vi "stacked secuence.vi"() -> ()   [LabVIEW 2020]
panel:
  out "Boolean":bool
  in  "Button":bool
  out "Thermometer":u8(slide) scale=0.0..100.0
  in  "stop":bool
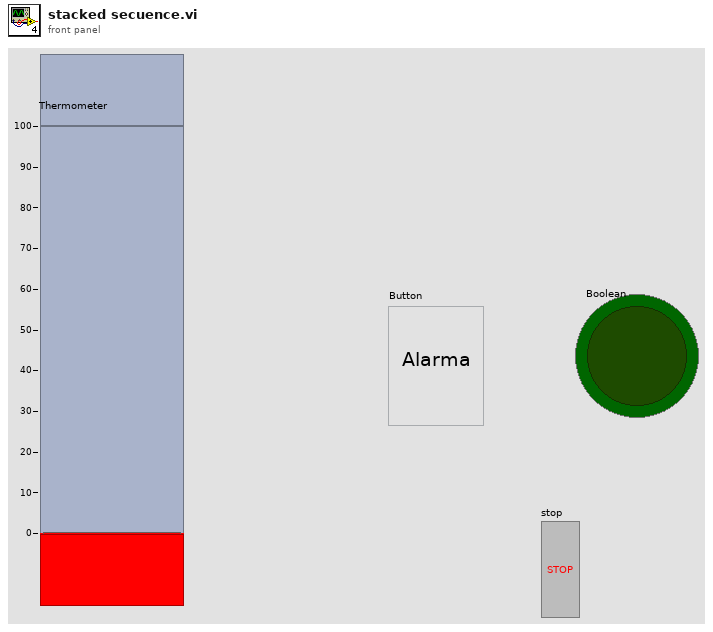
[diagram p1: front panel]
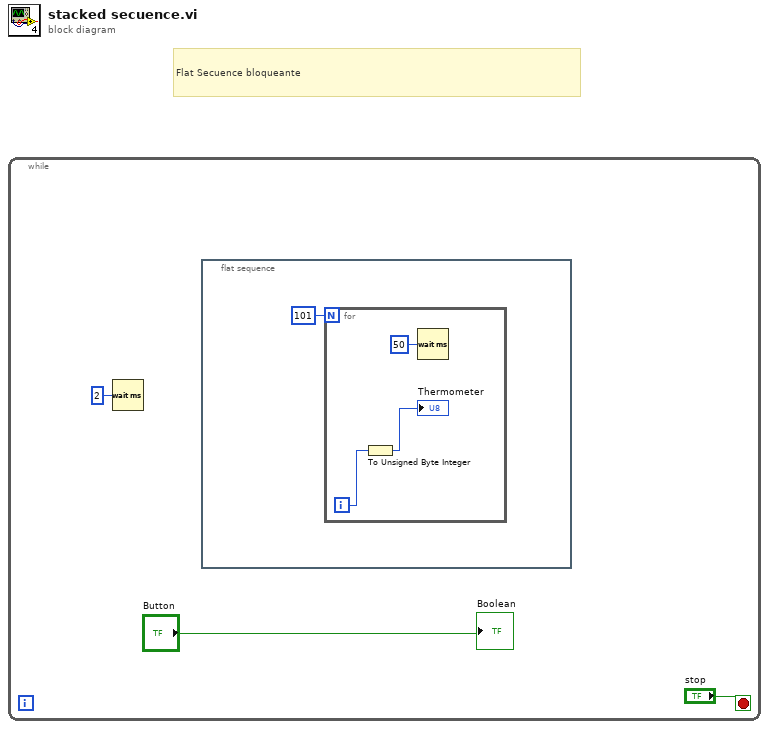
[diagram p0: block diagram]
diagram:
  # "Flat Secuence bloqueante"
  n1 = while {
    stop <- "stop" stop-if-true
    n2 = Wait (ms)(milliseconds to wait=u32 2) -> ()  [unwired: 1 out]
    n3 = flat-sequence {
      frame #0 {
        n4 = for {
          N: 101 -> [_]
          i -> [w7]
          n5 = To Unsigned Byte Integer(number=w7) -> (unsigned 8bit integer=→"Thermometer":u8)
          n6 = Wait (ms)(milliseconds to wait=u32 50) -> ()  [unwired: 1 out]
        }
      }
    }
    "Boolean" <- "Button"
  }
